vi "DAQ AI wo fgv.vi"(8 "error in":errorcluster, 10 "Config":T1={"min value"=-5.0, "max value"=5.0, "rate"=1000.0, "samples per channel"=100} {"rate" format="%#_13g"; "max value" format="%#_13g"; "min value" format="%#_13g"}, 11 "Channel":string) -> (0 "error out":errorcluster={"status"=TRUE, "code"=-200862, "source"="Property Node DAQmx Timing (arg 1) in DAQ AE.vi->Analog Input - Voltage and Thermocouple in a Single Task.vi <append>\n<B>Device: </B>DAQ_LO, DAQ_HI\n\n<B>Task Name: </B>_unnamedTask<42>"}, 3 "Data":dbl format="%0.2f")   [LabVIEW 2021]
uses:
  <vilib>/DAQmx/read.llb/DAQmx Read (Analog 1D DBL 1Chan NSamp).vi
  <vilib>/Analysis/baseanly.llb/Mean (DBL).vi
  <vilib>/DAQmx/create/channels.llb/DAQmx Create Channel (AI-Voltage-Basic).vi
  <vilib>/DAQmx/configure/timing.llb/DAQmx Timing (Sample Clock).vi
  <vilib>/DAQmx/miscellaneous.llb/DAQmx Fill In Error Info.vi
  <vilib>/Analysis/NI_AALBase.lvlib
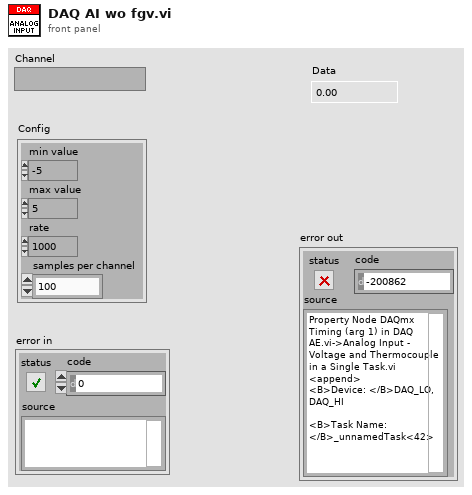
[diagram p1: front panel]
types:
  T1 = cluster{"min value":dbl, "max value":dbl, "rate":dbl, "samples per channel":i32}
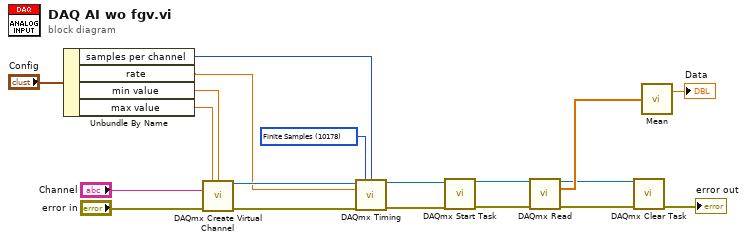
[diagram p0: block diagram]
diagram:
  w17 = 10178 items=["Finite Samples"=10178, "Continuous Samples"=10123, "Hardware Timed Single Point"=12522] ("sample mode")
  n1 = Unbundle By Name("Config") -> ("samples per channel"=w14:i32, "rate"=w13:dbl, "min value"=w2:dbl, "max value"=w1:dbl)
  n2 = call-poly <vilib>:"DAQmx Create Virtual Channel.vi"("maximum value"=w1, "minimum value"=w2, "physical channels"="Channel", "error in"="error in") -> ("task out"=w15:refnum<k21>, "error out"=w16:errorcluster)  [unwired: 10 in]
  n3 = call-poly <vilib>:"DAQmx Timing.vi"("task/channels in"=w15, "sample mode"=w17, "samples per channel"=w14, "rate"=w13, "error in"=w16) -> ("task out"=w10:refnum<k21>, "error out"=w11:errorcluster)  [unwired: 9 in]
  n4 = call <vilib>:"DAQmx Start Task.vi"("task/channels in"=w10, "error in"=w11) -> ("task out"=w9:refnum<k21>, "error out"=w12:errorcluster)  [unwired: 12 in]
  n5 = call-poly <vilib>:"DAQmx Read.vi"("task/channels in"=w9, "error in"=w12) -> ("task out"=w5:refnum<k21>, "data"=w7:dbl[], "error out"=w6:errorcluster)  [unwired: 11 in]
  n6 = call <vilib>:"DAQmx Clear Task.vi"("task in"=w5, "error in"=w6) -> ("error out"=→"error out":errorcluster)  [unwired: 13 in]
  n7 = call-poly <vilib>:"Mean.vi"("X"=w7) -> ("mean"=→"Data":dbl)  [unwired: 1 out]
